vi "VIght Light and Press Logic.vi"(0 "Score in":u16, 1 "Tick":i32, 2 "Debounce Threshold, ticks":u64, 3 "Speed Threshold, ticks":u64, 5 "Multiplier in":u16, 7 "Last Valid Press Tick in":u64, 9 "Debounce Tick in":u64[](array[numeric])=[0, 0, 0, 0, 0, 0, 0, 0, 0, 0, 0, 0, 0, 0, 0, 0, 0, 0, 0, 0], 11 "Lit Buttons":bool[](array[boolean])=[FALSE, FALSE, FALSE, FALSE, FALSE, FALSE, FALSE, FALSE, FALSE, FALSE, FALSE, FALSE, FALSE, FALSE, FALSE, FALSE, FALSE, FALSE, FALSE, FALSE], 12 "Pressed Buttons":bool[](array[boolean])=[FALSE, FALSE, FALSE, FALSE, FALSE, FALSE, FALSE, FALSE, FALSE, FALSE, FALSE, FALSE, FALSE, FALSE, FALSE, FALSE, FALSE, FALSE, FALSE, FALSE], 14 "Random Number":T1) -> (4 "Score out":u16, 6 "Multiplier out":u16, 8 "Last Valid Press Tick out":u64, 10 "Debounce Tick out":u64[](array[numeric]), 15 "Buttons to Light":bool[](array[boolean]))   [LabVIEW 2026]
uses:
  <extravilib>/ChannelInstances/Tag-u8/))Channel.ctl
  <vilib>/rvi/Emulation/niFpgaGetClockAttributes.vi
  <vilib>/rvi/Emulation/niFpgaSctlEmulationGetInTimedLoop.vi
  <vilib>/rvi/Emulation/niFpgaEmulationReportErrorSimple.vi
  <vilib>/rvi/Emulation/niFpgaCriticalErrorInLSC.vi
  <extravilib>/ChannelInstances/Tag-u8.lvlib
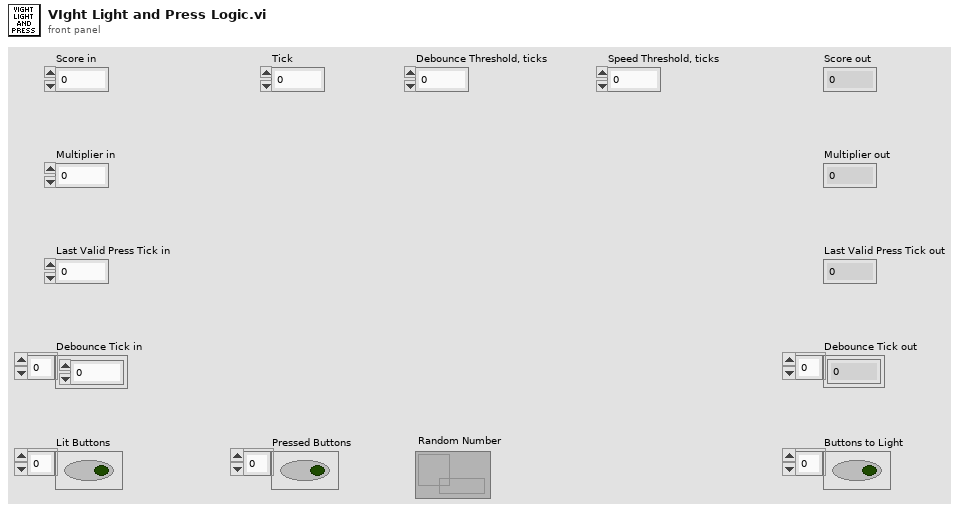
[diagram p1: front panel]
types:
  T1 = typedef "Tag-u8.lvlib/))Channel.ctl" = refnum<queue>
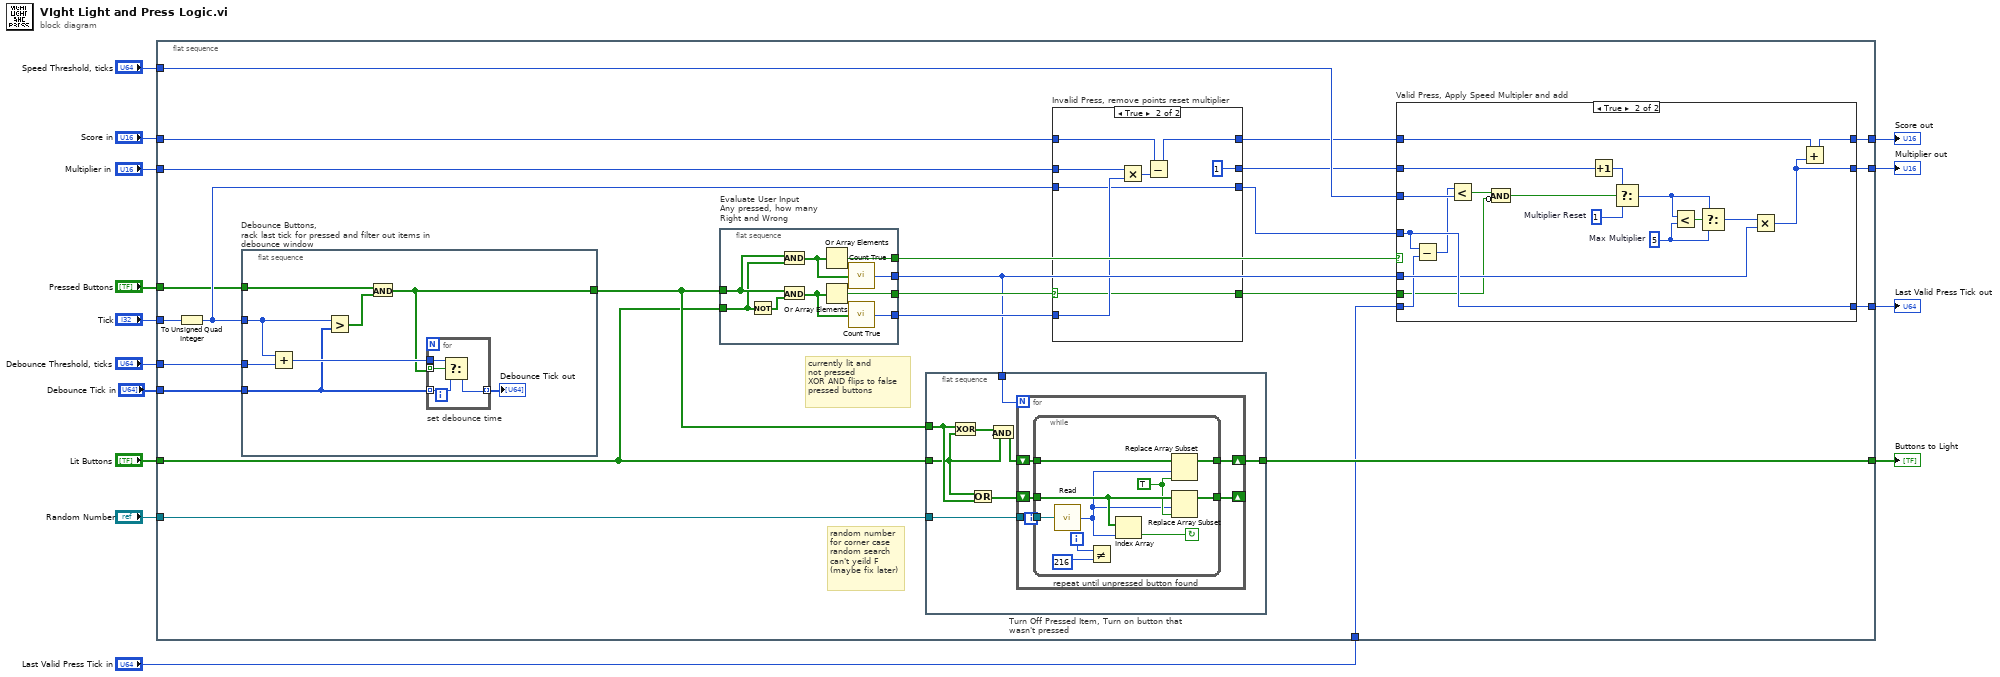
[diagram p0: block diagram]
diagram:
  n1 = flat-sequence {
    tunnel: "Tick" -> [w38]
    tunnel: "Debounce Threshold, ticks" -> [w37]
    tunnel: "Speed Threshold, ticks" -> [w36]
    tunnel: "Multiplier in" -> [w35]
    tunnel: "Score in" -> [w34]
    tunnel: [w26] -> w6
    tunnel: [w23] -> w7
    tunnel: [w22] -> w8
    tunnel: [w21] -> w9
    tunnel: "Lit Buttons" -> [w17]
    tunnel: "Last Valid Press Tick in" -> [w20]
    tunnel: "Pressed Buttons" -> [w18]
    tunnel: "Random Number" -> [w16]
    tunnel: "Debounce Tick in" -> [w15]
    frame #0 {
      # "random number\nfor corner case\nrandom search\ncan't yeild F\n(maybe fix later)"
      # "currently lit and \nnot pressed\nXOR AND flips to false \npressed buttons"
      n2 = To Unsigned Quad Integer(1:w38) -> (0:w28:u64)
      n3 = flat-sequence "Debounce Buttons, \nrack last tick for pressed and filter out items in debounce window" {
        tunnel: w37 -> [w67]
        tunnel: w28 -> [w66]
        tunnel: [w65] -> w24
        tunnel: w18 -> [w64]
        tunnel: w15 -> [w63]
        frame #0 {
          n4 = Add(x=w66, y=w67) -> (x+y=w68:u64)
          n5 = Greater?(x=w66, y=w63) -> (0:w69:bool[])
          n6 = And(x=w64, y=w69) -> (x .and. y?=w65:bool[])
          n7 = for "set debounce time" {
            tunnel: w65 -> [w73] mode=indexing
            tunnel: w63 -> [w71] mode=indexing
            tunnel: w68 -> [w72]
            tunnel: [w70] -> w62 mode=indexing
            n8 = Select(t=w72, s=w73, f=w71) -> (s? t:f=w70:u64)
          }
          "Debounce Tick out" <- w62
        }
      }
      n9 = flat-sequence "Evaluate User Input \nAny pressed, how many\nRight and Wrong" {
        tunnel: w24 -> [w82]
        tunnel: [w80] -> w32
        tunnel: w17 -> [w79]
        tunnel: [w78] -> w33
        tunnel: [w74] -> w31
        tunnel: [w76] -> w25
        frame #0 {
          n10 = Not(x=w79) -> (.not. x?=w81:bool[])
          n11 = And(x=w82, y=w79) -> (x .and. y?=w77:bool[])
          n12 = And(x=w82, y=w81) -> (x .and. y?=w75:bool[])
          n13 = Or Array Elements(Boolean array=w77) -> (logical OR=w78:bool)
          n14 = Or Array Elements(Boolean array=w75) -> (logical OR=w80:bool)
          n15 = call "Count True.vi"("Booleans"=w77) -> ("Count"=w76:u16)  [unwired: 14 in]
          n16 = call "Count True.vi"("Booleans"=w75) -> ("Count"=w74:u16)  [unwired: 14 in]
        }
      }
      n17 = flat-sequence "Turn Off Pressed Item, Turn on button that wasn't pressed" {
        tunnel: w24 -> [w42]
        tunnel: [w45] -> w22
        tunnel: w17 -> [w41]
        tunnel: w25 -> [w43]
        tunnel: w16 -> [w39]
        frame #0 {
          n18 = Exclusive Or(1:w41, 2:w42) -> (0:w46:bool[])
          n19 = Or(x=w41, y=w42) -> (x .or. y?=w40:bool[])
          n20 = And(x=w46, y=w41) -> (x .and. y?=w44:bool[])
          n21 = for {
            N: w43 -> [_]
            shift-right: [w50] -> w45
            shift-left: w44 -> [w51]
            shift-right: [w48] -> _
            shift-left: w40 -> [w49]
            tunnel: w39 -> [w47]
            n22 = while "repeat until unpressed button found" {
              tunnel: w51 -> [w61]
              tunnel: [w60] -> w50
              tunnel: w49 -> [w59]
              tunnel: [w58] -> w48
              tunnel: w47 -> [w52]
              i -> [w56]
              stop <- w54 continue-if-true
              w57 = TRUE ("new element/subarray")
              n23 = call <extravilib>:"Read.vi"("channel"=w52) -> ("element"=w53:u8)  [unwired: 1 in, 1 out]
              n24 = Not Equal?(x=w56, y=216 ("x")) -> ()  [unwired: 1 out]
              n25 = Index Array(array=w59, index=w53) -> (element=w54:bool)
              n26 = Replace Array Subset(array=w61, new element=w57, index=w53) -> (w60:bool[])
              n27 = Replace Array Subset(array=w59, new element=w57, index=w53) -> (w58:bool[])
            }
          }
        }
      }
      n28 = case "Invalid Press, remove points reset multiplier" shown="True" w32 {
        selector: w32 -> [w83 w89]
        tunnel: w35 -> [w86 w92]
        tunnel: w28 -> [w84 w87]
        tunnel: [w86 u16 1 ("Multiplier")] -> w29
        tunnel: w34 -> [w85 w93]
        tunnel: [w85 w94] -> w30
        tunnel: w31 -> [_ w91]
        tunnel: [w84 w87] -> w27
        tunnel: [w83 w89] -> w19
        frame False {
        }
        frame True {
          n29 = Multiply(x=w92, y=w91) -> (x*y=w90:u16)
          n30 = Subtract(x=w93, y=w90) -> (x-y=w94:u16)
        }
      }
      n31 = case "Valid Press, Apply Speed Multipler and add" shown="True" w33 {
        tunnel: w30 -> [w96 w114]
        tunnel: w29 -> [w97 w111]
        tunnel: [w97 w104] -> w21
        tunnel: [w96 w115] -> w23
        tunnel: w36 -> [_ w113]
        tunnel: [w95 w110] -> w26
        tunnel: w27 -> [_ w110]
        tunnel: w25 -> [_ w105]
        tunnel: w20 -> [w95 w100]
        tunnel: w19 -> [_ w98]
        frame False {
        }
        frame True {
          w108 = u16 5  # Max Multiplier
          w106 = u16 1  # Multiplier Reset
          n32 = Subtract(x=w110, y=w100) -> (x-y=w103:u64)
          n33 = Less?(x=w103, y=w113) -> (x < y?=w112:bool)
          n34 = Compound Arithmetic op=AND(w112, invert w98) -> (w99:bool)
          n35 = Increment(x=w111) -> (x+1=w107:u16)
          n36 = Select(t=w107, s=w99, f=w106) -> (s? t:f=w101:u16)
          n37 = Less?(x=w101, y=w108) -> (x < y?=w109:bool)
          n38 = Select(t=w101, s=w109, f=w108) -> (s? t:f=w102:u16)
          n39 = Multiply(x=w102, y=w105) -> (x*y=w104:u16)
          n40 = Add(x=w114, y=w104) -> (x+y=w115:u16)
        }
      }
    }
  }
  "Multiplier out" <- w9
  "Buttons to Light" <- w8
  "Score out" <- w7
  "Last Valid Press Tick out" <- w6
